vi "sftp_fstat.vi"() -> ()   [LabVIEW 2013]
doc: "Illustrates how to read and write file information by file descriptor."
uses:
  libssh2/libssh2_init_default.vi
  libssh2/libssh2_session_handshake_tcp.vi
  libssh2/libssh2.lvlib
panel:
  out "original mtime":timestamp
  out "new mtime":timestamp
  in  "file":string="/"
  out "error out":errorcluster
  in  "password":string
  in  "username":string
  in  "hostname":string
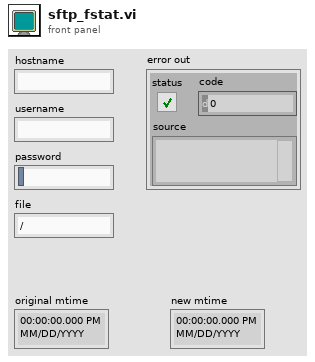
[diagram p1: front panel]
types:
  T1 = typedef "libssh2.lvlib/Session Refnum.ctl" = refnum<k1>
  T2 = typedef "libssh2.lvlib/SFTP Refnum.ctl" = refnum<k1>
  T3 = typedef "libssh2.lvlib/SFTP Handle Refnum.ctl" = refnum<k1>
  T4 = typedef "libssh2.lvlib/libssh2_sftp_attributes.ctl" = cluster{"flags":u32, "filesize":u64, "uid":u32, "gid":u32, "permissions":u32, "atime":u32, "mtime":u32}
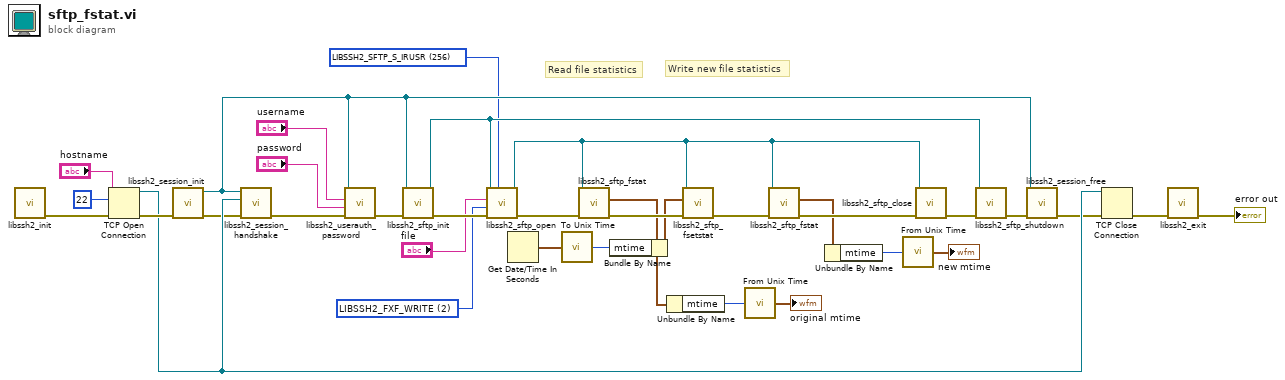
[diagram p0: block diagram]
diagram:
  w14 = u32 2 items=["LIBSSH2_FXF_READ"=1, "LIBSSH2_FXF_WRITE"=2, "LIBSSH2_FXF_APPEND"=4, "LIBSSH2_FXF_CREAT"=8, "LIBSSH2_FXF_TRUNC"=16, "LIBSSH2_FXF_EXCL"=32] ("flags")
  w15 = 256 items=["LIBSSH2_SFTP_S_IRWXU"=448, "LIBSSH2_SFTP_S_IRUSR"=256, "LIBSSH2_SFTP_S_IWUSR"=128, "LIBSSH2_SFTP_S_IXUSR"=64, "LIBSSH2_SFTP_S_IRWXG"=56, "LIBSSH2_SFTP_S_IRGRP"=32, "LIBSSH2_SFTP_S_IWGRP"=16, "LIBSSH2_SFTP_S_IXGRP"=8, "LIBSSH2_SFTP_S_IRWXO"=7, "LIBSSH2_SFTP_S_IROTH"=4, "LIBSSH2_SFTP_S_IWOTH"=2, "LIBSSH2_SFTP_S_IXOTH"=1] ("mode")
  # "Write new file statistics"
  # "Read file statistics"
  n1 = call-poly "libssh2_init.vi"() -> ("error out"=w34:errorcluster)  [unwired: 11 in]
  n2 = TCP Open Connection(address="hostname", remote port or service name=u16 22, error in (no error)=w34) -> (connection ID=w32:refnum<k5>, error out=w33:errorcluster)  [unwired: 2 in]
  n3 = call "libssh2_session_init.vi"("error in (no error)"=w33) -> ("error out"=w31:errorcluster, "session"=w24:T1)  [unwired: 9 in]
  n4 = call-poly "libssh2_session_handshake.vi"("error in (no error)"=w31, "tcp connection"=w32, "session"=w24) -> ("error out"=w35:errorcluster)  [unwired: 8 in]
  n5 = call "libssh2_userauth_password.vi"("error in (no error)"=w35, "password"="password", "username"="username", "session"=w24) -> ("error out"=w28:errorcluster)  [unwired: 7 in]
  n6 = call "libssh2_sftp_init.vi"("error in (no error)"=w28, "session"=w24) -> ("error out"=w20:errorcluster, "sftp"=w16:T2)  [unwired: 8 in]
  n7 = call "libssh2_sftp_open.vi"("mode"=w15, "error in (no error)"=w20, "flags"=w14, "path"="file", "sftp"=w16) -> ("error out"=w18:errorcluster, "sftp handle"=w8:T3)  [unwired: 5 in]
  n8 = Get Date/Time In Seconds() -> (seconds since 1Jan1904=w4:timestamp)
  n9 = call "To Unix Time.vi"("timestamp"=w4) -> ("unix time"=w5:u32)  [unwired: 1 in]
  n10 = call "libssh2_sftp_fstat.vi"("error in (no error)"=w18, "sftp handle"=w8) -> ("error out"=w19:errorcluster, "attributes out"=w1:T4)  [unwired: 8 in]
  n11 = Bundle By Name(cluster=w1, "mtime"=w5) -> (w6:T4)
  n12 = Unbundle By Name(w1) -> ("mtime"=w2:u32)
  n13 = call "libssh2_sftp_fsetstat.vi"("error in (no error)"=w19, "attributes"=w6, "sftp handle"=w8) -> ("error out"=w10:errorcluster)  [unwired: 8 in]
  n14 = call "From Unix Time.vi"("unix time"=w2) -> ("timestamp"=→"original mtime":timestamp)  [unwired: 1 in]
  n15 = call "libssh2_sftp_fstat.vi"("error in (no error)"=w10, "sftp handle"=w8) -> ("error out"=w9:errorcluster, "attributes out"=w7:T4)  [unwired: 8 in]
  n16 = Unbundle By Name(w7) -> ("mtime"=w12:u32)
  n17 = call "From Unix Time.vi"("unix time"=w12) -> ("timestamp"=→"new mtime":timestamp)  [unwired: 1 in]
  n18 = call "libssh2_sftp_close.vi"("error in (no error)"=w9, "sftp handle"=w8) -> ("error out"=w13:errorcluster)  [unwired: 9 in]
  n19 = call "libssh2_sftp_shutdown.vi"("error in (no error)"=w13, "sftp"=w16) -> ("error out"=w21:errorcluster)  [unwired: 9 in]
  n20 = call "libssh2_session_free.vi"("error in (no error)"=w21, "session"=w24) -> ("error out"=w23:errorcluster)  [unwired: 9 in]
  n21 = TCP Close Connection(connection ID=w32, error in (no error)=w23) -> (error out=w22:errorcluster)  [unwired: 1 in, 1 out]
  n22 = call "libssh2_exit.vi"("error in (no error)"=w22) -> ("error out"=→"error out":errorcluster)  [unwired: 10 in]
